vi "FreqToPB.vi"(0 "Input Frequency [MHz]":dbl min=0.0 max=159.9999999 step=1.0000000000287557e-07 format="%.7g") -> (1 "PB Output Bits":bool[](array[boolean]), 2 "PB Output Value":u32 format="%06x")   [LabVIEW 2013, in "PTS-via-PB.lvclass"]
uses:
  PTS-via-PB.lvclass
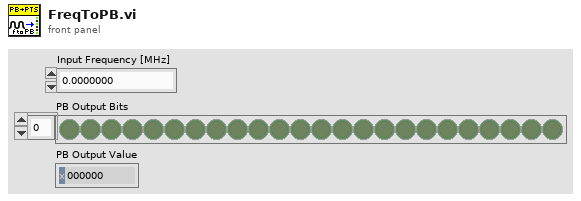
[diagram p1: front panel]
types:
  T1 = cluster{"8: 10 MHz":bool, "4: 10 MHz":bool, "2: 10 MHz":bool, "1: 10 MHz":bool, "8: 1 MHz":bool, "4: 1 MHz":bool, "2: 1 MHz":bool, "1: 1 MHz":bool, "8: 100 kHz":bool, "4: 100 kHz":bool, "2: 100 kHz":bool, "1: 100 kHz":bool, "8: 10 kHz":bool, "4: 10 kHz":bool, "2: 10 kHz":bool, "1: 10 kHz":bool, "8: 1 kHz":bool, "4: 1 kHz":bool, "2: 1 kHz":bool, "1: 1 kHz":bool, "8: 100 Hz":bool, "4: 100 Hz":bool, "2: 100 Hz":bool, "1: 100 Hz":bool, "8: 10 Hz":bool, "4: 10 Hz":bool, "2: 10 Hz":bool, "1: 10 Hz":bool, "8: 1 Hz":bool, "4: 1 Hz":bool, "2: 1 Hz":bool, "1: 1 Hz":bool, "8: 0.1 Hz":bool, "4: 0.1 Hz":bool, "2: 0.1 Hz":bool, "1: 0.1 Hz":bool}
  T2 = cluster{"[0]":bool, "[1]":bool, "[2]":bool, "[3]":bool, "[4]":bool, "[5]":bool, "[6]":bool, "[7]":bool, "[8]":bool, "[9]":bool, "[10]":bool, "[11]":bool, "[12]":bool, "[13]":bool, "[14]":bool, "[15]":bool, "[16]":bool, "[17]":bool, "[18]":bool, "[19]":bool, "[20]":bool, "[21]":bool, "[22]":bool, "[23]":bool, "[24]":bool, "[25]":bool, "[26]":bool, "[27]":bool, "[28]":bool, "[29]":bool, "[30]":bool, "[31]":bool, "[32]":bool, "[33]":bool, "[34]":bool, "[35]":bool}
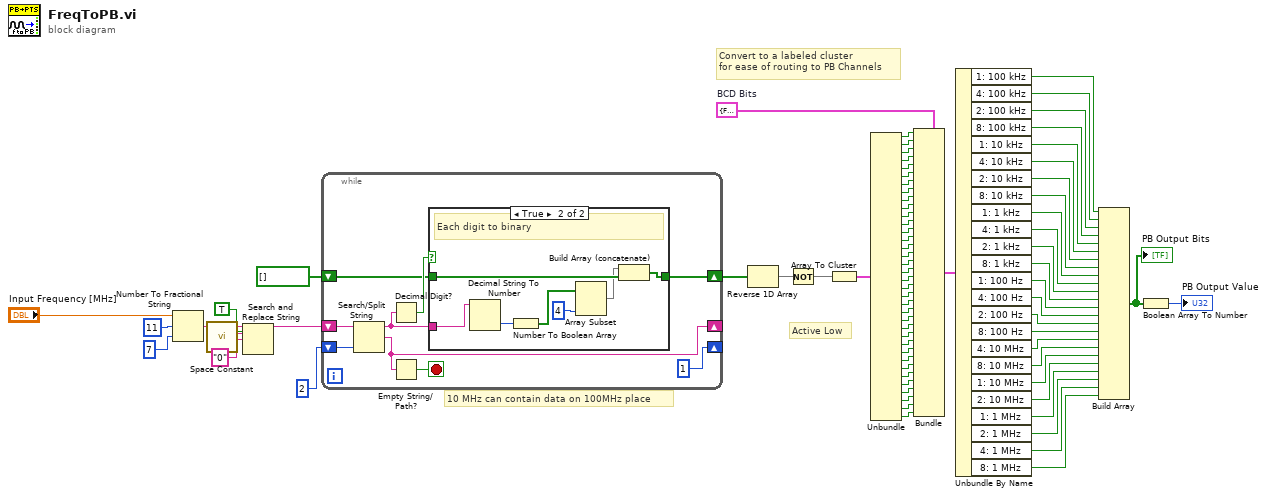
[diagram p0: block diagram]
diagram:
  w78 = T1 {"8: 10 MHz"=FALSE, "4: 10 MHz"=FALSE, "2: 10 MHz"=FALSE, "1: 10 MHz"=FALSE, "8: 1 MHz"=FALSE, "4: 1 MHz"=FALSE, "2: 1 MHz"=FALSE, "1: 1 MHz"=FALSE, "8: 100 kHz"=FALSE, "4: 100 kHz"=FALSE, "2: 100 kHz"=FALSE, "1: 100 kHz"=FALSE, "8: 10 kHz"=FALSE, "4: 10 kHz"=FALSE, "2: 10 kHz"=FALSE, "1: 10 kHz"=FALSE, "8: 1 kHz"=FALSE, "4: 1 kHz"=FALSE, "2: 1 kHz"=FALSE, "1: 1 kHz"=FALSE, "8: 100 Hz"=FALSE, "4: 100 Hz"=FALSE, "2: 100 Hz"=FALSE, "1: 100 Hz"=FALSE, "8: 10 Hz"=FALSE, "4: 10 Hz"=FALSE, "2: 10 Hz"=FALSE, "1: 10 Hz"=FALSE, "8: 1 Hz"=FALSE, "4: 1 Hz"=FALSE, "2: 1 Hz"=FALSE, "1: 1 Hz"=FALSE, "8: 0.1 Hz"=FALSE, "4: 0.1 Hz"=FALSE, "2: 0.1 Hz"=FALSE, "1: 0.1 Hz"=FALSE}  # BCD Bits
  # "10 MHz can contain data on 100MHz place"
  # "Active Low"
  # "Convert to a labeled cluster\nfor ease of routing to PB Channels"
  n1 = Number To Fractional String(number="Input Frequency [MHz]", width (-)=i16 11, precision (6)=i16 7) -> (F-format string=w35:string)  [unwired: 1 in]
  n2 = call <vilib>:"Space Constant.vi"() -> ("String"=w34:string)
  n3 = Search and Replace String(replace all?=TRUE ("replace all? (F)"), input string=w35, search string=w34, replace string="0" ("replace string (\"\")")) -> (result string=w31:string)  [unwired: 4 in, 3 out]
  n4 = while {
    shift-right: [w83] -> _
    shift-left: w31 -> [w87]
    shift-right: [1] -> _
    shift-left: 2 -> [w86]
    shift-right: [w80] -> w28
    shift-left: bool[] [] -> [w79]
    stop <- w85 stop-if-true
    n5 = Search/Split String(string=w87, offset (0)=w86) -> (substring before match=w81:string, match + rest of string=w83:string)  [unwired: 1 in, 1 out]
    n6 = Decimal Digit?(1:w81) -> (0:w82:bool)
    n7 = Empty String/Path?(string/path=w83) -> (empty?=w85:bool)
    n8 = case shown="True" w82 {
      tunnel: w81 -> [_ w92]
      tunnel: [w88 w94] -> w80
      tunnel: w79 -> [w88 w93]
      frame False {
        # "Skip decimal decoding"
      }
      frame True {
        # "Each digit to binary"
        n9 = Decimal String To Number(string=w92) -> (number=w91:i32)  [unwired: 2 in, 1 out]
        n10 = Number To Boolean Array(number=w91) -> (Boolean array=w90:bool[])
        n11 = Array Subset(array=w90, length=4) -> (w89:bool[])  [unwired: 1 in]
        n12 = Build Array (concatenate)(w89, w93) -> (w94:bool[])
      }
    }
  }
  n13 = Reverse 1D Array(array=w28) -> (reversed array=w27:bool[])
  n14 = Not(x=w27) -> (.not. x?=w39:bool[])
  n15 = Array To Cluster(array=w39) -> (cluster=w77:T2)
  n16 = Unbundle(w77) -> ("[0]"=w76:bool, "[1]"=w75:bool, "[2]"=w74:bool, "[3]"=w73:bool, "[4]"=w72:bool, "[5]"=w71:bool, "[6]"=w70:bool, "[7]"=w69:bool, "[8]"=w68:bool, "[9]"=w67:bool, "[10]"=w66:bool, "[11]"=w65:bool, "[12]"=w64:bool, "[13]"=w63:bool, "[14]"=w62:bool, "[15]"=w61:bool, "[16]"=w60:bool, "[17]"=w59:bool, "[18]"=w58:bool, "[19]"=w57:bool, "[20]"=w56:bool, "[21]"=w55:bool, "[22]"=w54:bool, "[23]"=w53:bool, "[24]"=w52:bool, "[25]"=w51:bool, "[26]"=w50:bool, "[27]"=w49:bool, "[28]"=w48:bool, "[29]"=w47:bool, "[30]"=w46:bool, "[31]"=w45:bool, "[32]"=w44:bool, "[33]"=w43:bool, "[34]"=w42:bool, "[35]"=w41:bool)
  n17 = Bundle(cluster=w78, "8: 10 MHz"=w76, "4: 10 MHz"=w75, "2: 10 MHz"=w74, "1: 10 MHz"=w73, "8: 1 MHz"=w72, "4: 1 MHz"=w71, "2: 1 MHz"=w70, "1: 1 MHz"=w69, "8: 100 kHz"=w68, "4: 100 kHz"=w67, "2: 100 kHz"=w66, "1: 100 kHz"=w65, "8: 10 kHz"=w64, "4: 10 kHz"=w63, "2: 10 kHz"=w62, "1: 10 kHz"=w61, "8: 1 kHz"=w60, "4: 1 kHz"=w59, "2: 1 kHz"=w58, "1: 1 kHz"=w57, "8: 100 Hz"=w56, "4: 100 Hz"=w55, "2: 100 Hz"=w54, "1: 100 Hz"=w53, "8: 10 Hz"=w52, "4: 10 Hz"=w51, "2: 10 Hz"=w50, "1: 10 Hz"=w49, "8: 1 Hz"=w48, "4: 1 Hz"=w47, "2: 1 Hz"=w46, "1: 1 Hz"=w45, "8: 0.1 Hz"=w44, "4: 0.1 Hz"=w43, "2: 0.1 Hz"=w42, "1: 0.1 Hz"=w41) -> (w40:T1)
  n18 = Unbundle By Name(w40) -> ("1: 100 kHz"=w26:bool, "4: 100 kHz"=w25:bool, "2: 100 kHz"=w24:bool, "8: 100 kHz"=w23:bool, "1: 10 kHz"=w22:bool, "4: 10 kHz"=w21:bool, "2: 10 kHz"=w20:bool, "8: 10 kHz"=w19:bool, "1: 1 kHz"=w18:bool, "4: 1 kHz"=w17:bool, "2: 1 kHz"=w16:bool, "8: 1 kHz"=w15:bool, "1: 100 Hz"=w14:bool, "4: 100 Hz"=w13:bool, "2: 100 Hz"=w12:bool, "8: 100 Hz"=w11:bool, "4: 10 MHz"=w10:bool, "8: 10 MHz"=w9:bool, "1: 10 MHz"=w8:bool, "2: 10 MHz"=w7:bool, "1: 1 MHz"=w6:bool, "2: 1 MHz"=w5:bool, "4: 1 MHz"=w4:bool, "8: 1 MHz"=w3:bool)
  n19 = Build Array(w26, w25, w24, w23, w22, w21, w20, w19, w18, w17, w16, w15, w14, w13, w12, w11, w10, w9, w8, w7, w6, w5, w4, w3) -> (w2:bool[])
  "PB Output Bits" <- w2
  n20 = Boolean Array To Number(Boolean array=w2) -> (number=→"PB Output Value":u32)
